vi "IO输入界面.vi"(8 "错误输入（无错误）":errorcluster, 10 "界面切换队列":refnum<queue>, 11 "VISA资源名称输入":refnum<visa-resource-name>) -> (0 "错误输出":errorcluster, 3 "VISA资源名称输出":refnum<visa-resource-name>)   [LabVIEW 2018]
panel:
  out "毫秒计时值":u32
  in  "枚举":T1(ring)
  in  "选项卡控件":enum32{"选项卡 1", "选项卡 2"}(tab)
  out "IO输出":bool
  out "X308-9#OK":bool
  out "?":bool
  out "?":bool
  out "X207-16#正在烧录":bool
  out "X206-15#正在烧录":bool
  out "X205-14#正在烧录":bool
  out "X204-13#正在烧录":bool
  out "X203-12#正在烧录":bool
  out "X202-11#正在烧录":bool
  out "X201-10#正在烧录":bool
  out "X200-9#正在烧录":bool
  out "X317-8#正在烧录":bool
  out "X316-7#正在烧录":bool
  out "X315-6#正在烧录":bool
  out "X314-5#正在烧录":bool
  out "X313-4#正在烧录":bool
  out "X312-3#正在烧录":bool
  out "X311-2#正在烧录":bool
  out "X310-1#正在烧录":bool
  out "X30F-16#OK":bool
  out "X30E-15#OK":bool
  out "X30D-14#OK":bool
  out "X30C-13#OK":bool
  out "X30B-12#OK":bool
  out "X30A-11#OK":bool
  out "X309-10#OK":bool
  out "X307-8#OK":bool
  out "X306-7#OK":bool
  out "X305-6#OK":bool
  out "X304-5#OK":bool
  out "X303-4#OK":bool
  out "X302-3#OK":bool
  out "X301-2#OK":bool
  out "X300-1#OK":bool
  out "X1F-Z2轴伺服报警":bool
  out "X1E-Z1轴伺服报警":bool
  out "X1D-Y轴伺服报警":bool
  out "X1C-X轴伺服报警":bool
  out "X1B":bool
  out "X1A":bool
  out "X19":bool
  out "X18":bool
  out "X17-2号真空达到":bool
  out "X16-1号真空到达":bool
  out "X15-手柄快慢切换":bool
  out "X14手柄Z1+":bool
  out "X13-手柄Z1-":bool
  out "X12-手柄X-":bool
  out "X11-手柄X+":bool
  out "X10-手柄Y+":bool
  out "XF-手柄Y-":bool
  out "XE":bool
  out "XD":bool
  out "XC-自动换盘完成":bool
  out "XB-卷带收料完成":bool
  out "XA-启动按钮":bool
  out "X9-紧急停止":bool
  out "X8-开门检测":bool
  out "X7-Z2原点":bool
  out "X6-Z1原点":bool
  out "X5-Y轴原点":bool
  out "X4-X轴原点":bool
  out "X3":bool
  out "X2":bool
  out "X1":bool
  out "DDT90356":dbl
  out "DDT90348":dbl
  out "自动界面":bool
  out "手动界面":bool
  out "参数界面":bool
  out "IO界面":bool
  out "产品界面":bool
  out "字符串":string
  out "DDT90352":dbl
  out "DDT90360":dbl
  out "通讯周期":dbl
  out "DT1184":T2(ring)
  out "X0":bool
  # "X"
  # "Z1"
  # "XXXXX自动化设备有限公司"
  # "Z2"
  # "Y"
  # "本\n体\n输\n入"
  # "扩\n展\n输\n入"
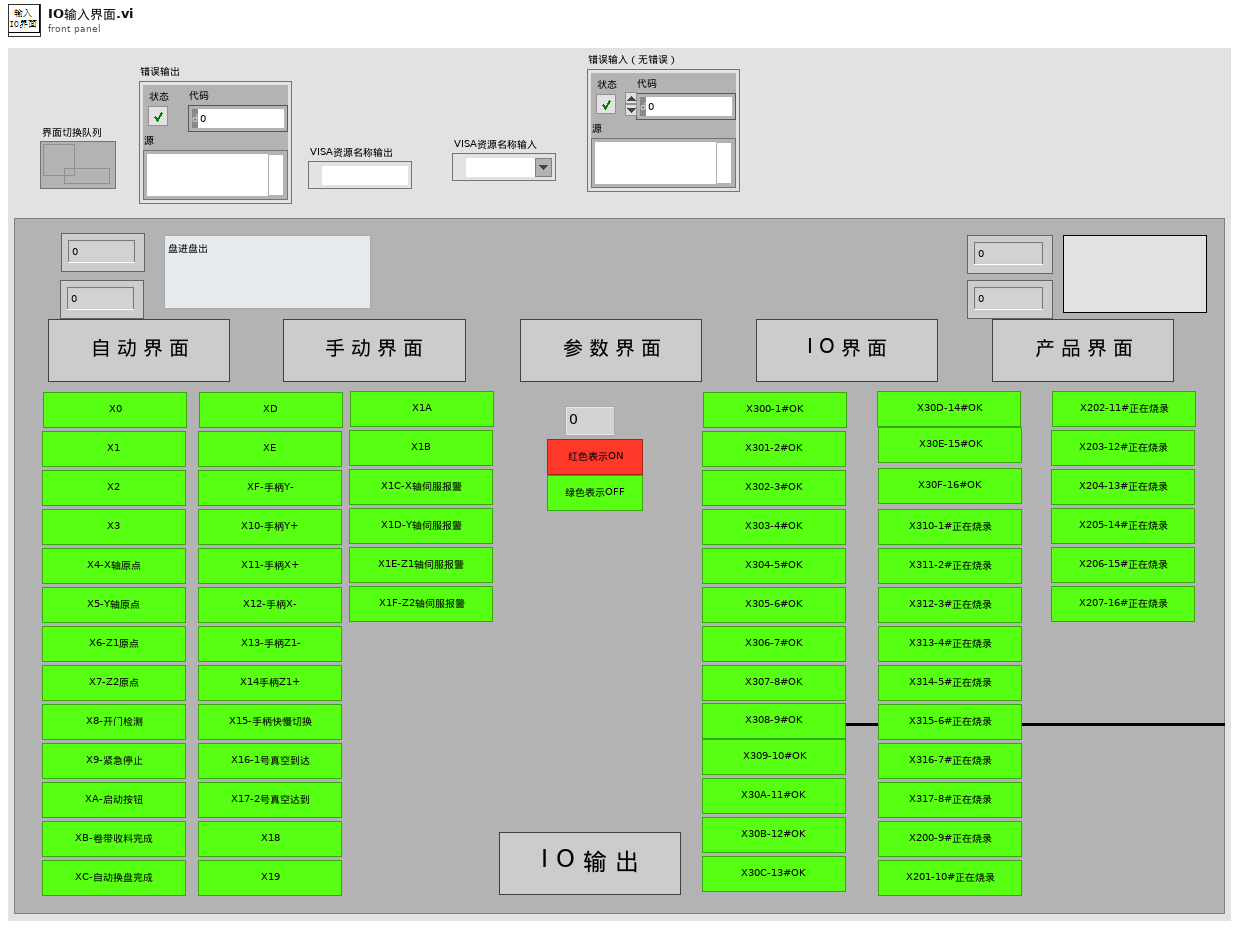
[diagram p1: front panel]
types:
  T1 = enum16{"读初始化", "读X310+8", "读X200+8", "读X308+8", "读X300+8", "读X18+8", "读X10+8", "读X8+8", "读X0+8", "读DDT90356", "读DT1184", "读DDT90348", ""}
  T2 = enum16{"盘进盘出", "卷进卷出", "盘进卷出", "管进盘出", "管进卷出", "卷进盘出", ""}
  T3 = enum8{"Enabled", "Disabled", "Disabled and Grayed Out"}
  T4 = typedef "数据簇.ctl" = cluster{"字符串":string, "数值":i32, "布尔":bool}
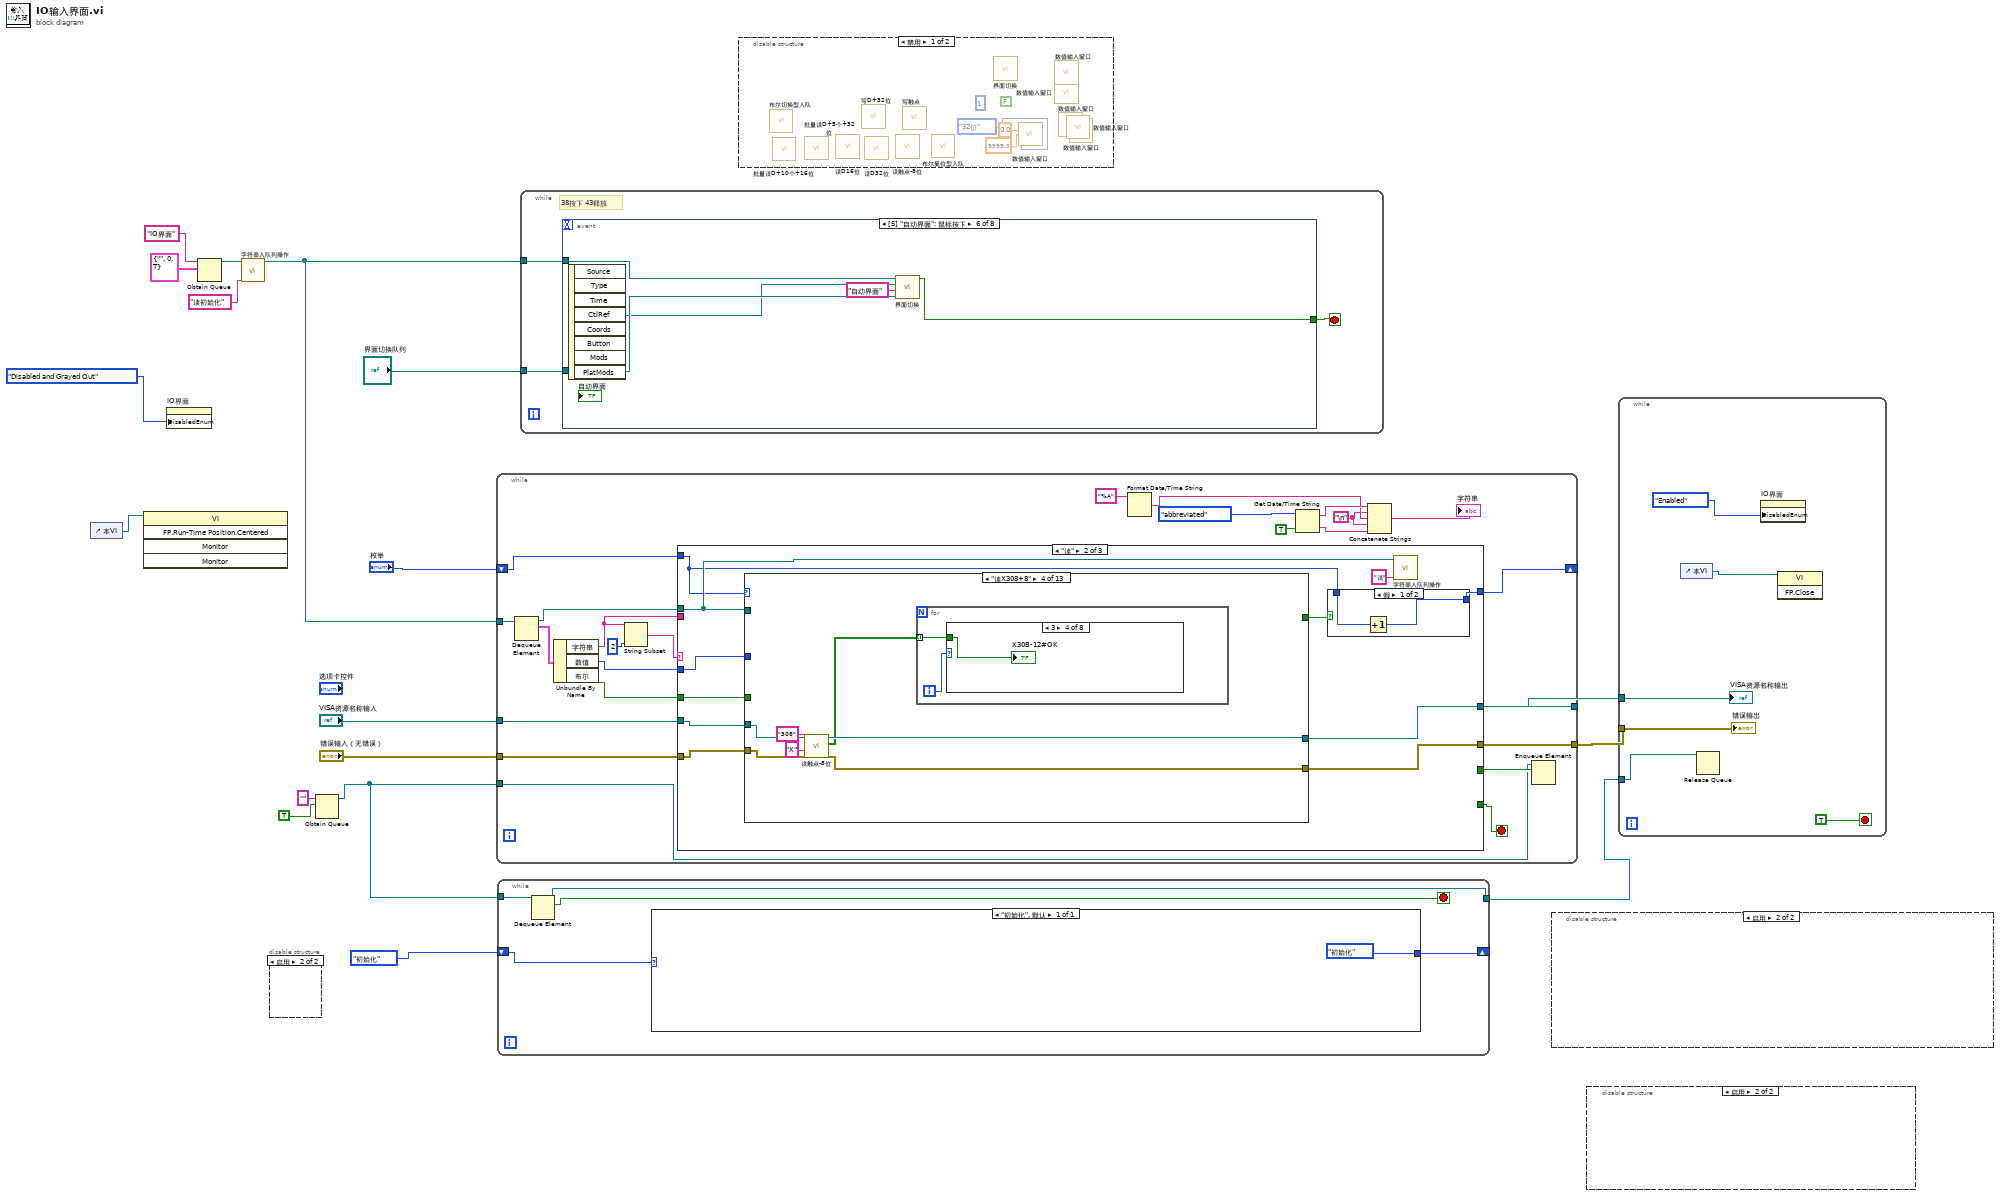
[diagram p0: block diagram]
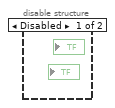
[diagram p2: hidden frame]
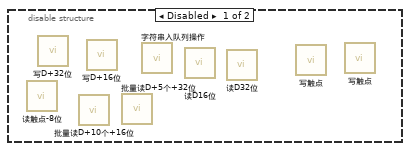
[diagram p20: hidden frame]
diagram:
  n1 = control-ref of="本VI"() -> (w1:refnum<vi>)
  n2 = invoke class="VI" method="FP.Run-Time Position.Centered"(reference=w1) -> ()  [unwired: 4 in, 5 out]
  n3 = property on="IO界面" class="Bool"("DisabledEnum"=T3."Disabled and Grayed Out" ("禁用")) -> ()  [unwired: 2 in, 2 out]
  n4 = Obtain Queue(name (unnamed)="IO界面" ("名称（未命名）"), element data type=T4 {"字符串"="", "数值"=0, "布尔"=TRUE}) -> (queue out=w11:refnum<queue>)  [unwired: 3 in, 2 out]
  n5 = call "字符串入队列操作.vi"("字符消息入队列"="读初始化", "界面切换队列"=w11) -> ("队列输出"=w3:refnum<queue>)  [unwired: 9 in]
  n6 = disable-structure shown="启用" {
    frame Disabled {
    }
    frame Enabled {
    }
  }
  n7 = Obtain Queue(name (unnamed)="" ("名称（未命名）"), element data type=TRUE) -> (queue out=w6:refnum<queue>)  [unwired: 3 in, 2 out]
  n8 = while {
    tunnel: w3 -> [w39]
    tunnel: "VISA资源名称输入" -> [w32]
    tunnel: "错误输入（无错误）" -> [w31]
    tunnel: [w30] -> w13
    tunnel: [w29] -> w12
    shift-right: [w26] -> _
    shift-left: "枚举" -> [w27]
    tunnel: w6 -> [w19]
    stop <- w21 stop-if-true
    w23 = "\n"
    n9 = Dequeue Element(queue=w39) -> (queue out=w36:refnum<queue>, element=w38:T4)  [unwired: 2 in, 2 out]
    n10 = Unbundle By Name(w38) -> ("字符串"=w33:string, "数值"=w35:i32, "布尔"=w34:bool)
    n11 = String Subset(string=w33, length (rest)=2 ("长度（剩余）")) -> (substring=w37:string)  [unwired: 1 in]
    n12 = case shown="\"读\"" w37 {
      selector: w37 -> [w46 _ _]
      tunnel: w36 -> [_ w54 w259]
      tunnel: w35 -> [_ w61 w258]
      tunnel: w34 -> [_ w60 w257]
      tunnel: w33 -> [_ _ w251]
      tunnel: w32 -> [w45 w59 w256]
      tunnel: w31 -> [w44 w58 w255]
      tunnel: [w45 w57 w253] -> w30
      tunnel: [w44 w56 w252] -> w29
      tunnel: [_ _ w254] -> w21
      tunnel: w27 -> [_ w52 _]
      tunnel: [_ w51 _] -> w26
      tunnel: [_ _ w249] -> w20
      frame "", Default {
        n13 = Concatenate Strings("无对应消息分支**" ("消息"), w46, "**" ("字符串"), "读写状态机" ("字符串")) -> (w48:string)
        n14 = One Button Dialog(message=w48) -> ()  [unwired: 1 in, 1 out]
      }
      frame "读" {
        n15 = case shown="\"读X308+8\"" w52 {
          tunnel: w54 -> [_ _ _ _ _ _ _ _ _ _ _ _ _]
          tunnel: w61 -> [_ _ _ _ _ _ _ _ _ _ _ _ _]
          tunnel: w59 -> [w66 w73 w90 w107 w124 w141 w158 w175 w192 w214 w223 w236 w248]
          tunnel: w58 -> [w65 w72 w89 w106 w123 w140 w157 w174 w191 w213 w222 w235 w247]
          tunnel: [w66 w69 w86 w103 w120 w139 w154 w171 w190 w212 w221 w234 w248] -> w57
          tunnel: [w65 w68 w85 w102 w119 w138 w153 w170 w189 w211 w220 w233 w247] -> w56
          tunnel: w60 -> [_ _ _ _ _ _ _ _ _ _ _ _ _]
          tunnel: [_ _ _ _ _ _ _ _ _ _ _ _ TRUE] -> w53
          frame "读初始化" {
            n16 = Tick Count (ms)() -> (millisecond timer value=→"毫秒计时值":u32)
          }
          frame "读X310+8" {
            n17 = call "读触点-8位.vi"("error out"=w72, "触点类型"="X", "读取起始地址"="310", "VISA resource name out"=w73) -> ("error IO"=w68:errorcluster, "读取布尔数组"=w67:bool[], "VISA resource name out 2"=w69:refnum<visa-resource-name>)  [unwired: 4 in, 1 out]
            n18 = for {
              tunnel: w67 -> [w74] mode=indexing
              i -> [w75]
              n19 = case shown="7" w75 {
                tunnel: w74 -> [w76 w77 w78 w79 w80 w81 w82 w83]
                frame 0, Default {
                  "X310-1#正在烧录" <- w76
                }
                frame 1 {
                  "X311-2#正在烧录" <- w77
                }
                frame 2 {
                  "X312-3#正在烧录" <- w78
                }
                frame 3 {
                  "X313-4#正在烧录" <- w79
                }
                frame 4 {
                  "X314-5#正在烧录" <- w80
                }
                frame 5 {
                  "X315-6#正在烧录" <- w81
                }
                frame 6 {
                  "X316-7#正在烧录" <- w82
                }
                frame 7 {
                  "X317-8#正在烧录" <- w83
                }
              }
            }
          }
          frame "读X200+8" {
            n20 = call "读触点-8位.vi"("error out"=w89, "触点类型"="X", "读取起始地址"="200", "VISA resource name out"=w90) -> ("error IO"=w85:errorcluster, "读取布尔数组"=w84:bool[], "VISA resource name out 2"=w86:refnum<visa-resource-name>)  [unwired: 4 in, 1 out]
            n21 = for {
              tunnel: w84 -> [w91] mode=indexing
              i -> [w92]
              n22 = case shown="7" w92 {
                tunnel: w91 -> [w93 w94 w95 w96 w97 w98 w99 w100]
                frame 0, Default {
                  "X200-9#正在烧录" <- w93
                }
                frame 1 {
                  "X201-10#正在烧录" <- w94
                }
                frame 2 {
                  "X202-11#正在烧录" <- w95
                }
                frame 3 {
                  "X203-12#正在烧录" <- w96
                }
                frame 4 {
                  "X204-13#正在烧录" <- w97
                }
                frame 5 {
                  "X205-14#正在烧录" <- w98
                }
                frame 6 {
                  "X206-15#正在烧录" <- w99
                }
                frame 7 {
                  "X207-16#正在烧录" <- w100
                }
              }
            }
          }
          frame "读X308+8" {
            n23 = call "读触点-8位.vi"("error out"=w106, "触点类型"="X", "读取起始地址"="308", "VISA resource name out"=w107) -> ("error IO"=w102:errorcluster, "读取布尔数组"=w101:bool[], "VISA resource name out 2"=w103:refnum<visa-resource-name>)  [unwired: 4 in, 1 out]
            n24 = for {
              tunnel: w101 -> [w108] mode=indexing
              i -> [w109]
              n25 = case shown="3" w109 {
                tunnel: w108 -> [w110 w111 w112 w113 w114 w115 w116 w117]
                frame 0, Default {
                  "X308-9#OK" <- w110
                }
                frame 1 {
                  "X309-10#OK" <- w111
                }
                frame 2 {
                  "X30A-11#OK" <- w112
                }
                frame 3 {
                  "X30B-12#OK" <- w113
                }
                frame 4 {
                  "X30C-13#OK" <- w114
                }
                frame 5 {
                  "X30D-14#OK" <- w115
                }
                frame 6 {
                  "X30E-15#OK" <- w116
                }
                frame 7 {
                  "X30F-16#OK" <- w117
                }
              }
            }
          }
          frame "读X300+8" {
            n26 = call "读触点-8位.vi"("error out"=w123, "触点类型"="X", "读取起始地址"="300", "VISA resource name out"=w124) -> ("error IO"=w119:errorcluster, "读取布尔数组"=w118:bool[], "VISA resource name out 2"=w120:refnum<visa-resource-name>)  [unwired: 4 in, 1 out]
            n27 = for {
              tunnel: w118 -> [w125] mode=indexing
              i -> [w126]
              n28 = case shown="7" w126 {
                tunnel: w125 -> [w127 w128 w129 w130 w131 w132 w133 w134]
                frame 0, Default {
                  "X300-1#OK" <- w127
                }
                frame 1 {
                  "X301-2#OK" <- w128
                }
                frame 2 {
                  "X302-3#OK" <- w129
                }
                frame 3 {
                  "X303-4#OK" <- w130
                }
                frame 4 {
                  "X304-5#OK" <- w131
                }
                frame 5 {
                  "X305-6#OK" <- w132
                }
                frame 6 {
                  "X306-7#OK" <- w133
                }
                frame 7 {
                  "X307-8#OK" <- w134
                }
              }
            }
          }
          frame "读X18+8" {
            n29 = call "读触点-8位.vi"("error out"=w140, "触点类型"="X", "读取起始地址"="18", "VISA resource name out"=w141) -> ("error IO"=w138:errorcluster, "读取布尔数组"=w135:bool[], "VISA resource name out 2"=w139:refnum<visa-resource-name>)  [unwired: 4 in, 1 out]
            n30 = for {
              tunnel: w135 -> [w142] mode=indexing
              i -> [w143]
              n31 = case shown="7" w143 {
                tunnel: w142 -> [w144 w145 w146 w147 w148 w149 w150 w151]
                frame 0, Default {
                  "X18" <- w144
                }
                frame 1 {
                  "X19" <- w145
                }
                frame 2 {
                  "X1A" <- w146
                }
                frame 3 {
                  "X1B" <- w147
                }
                frame 4 {
                  "X1C-X轴伺服报警" <- w148
                }
                frame 5 {
                  "X1D-Y轴伺服报警" <- w149
                }
                frame 6 {
                  "X1E-Z1轴伺服报警" <- w150
                }
                frame 7 {
                  "X1F-Z2轴伺服报警" <- w151
                }
              }
            }
          }
          frame "读X10+8" {
            n32 = call "读触点-8位.vi"("error out"=w157, "触点类型"="X", "读取起始地址"="10", "VISA resource name out"=w158) -> ("error IO"=w153:errorcluster, "读取布尔数组"=w152:bool[], "VISA resource name out 2"=w154:refnum<visa-resource-name>)  [unwired: 4 in, 1 out]
            n33 = for {
              tunnel: w152 -> [w159] mode=indexing
              i -> [w160]
              n34 = case shown="0, 默认" w160 {
                tunnel: w159 -> [w161 w162 w163 w164 w165 w166 w167 w168]
                frame 0, Default {
                  "X10-手柄Y+" <- w161
                }
                frame 1 {
                  "X11-手柄X+" <- w162
                }
                frame 2 {
                  "X12-手柄X-" <- w163
                }
                frame 3 {
                  "X13-手柄Z1-" <- w164
                }
                frame 4 {
                  "X14手柄Z1+" <- w165
                }
                frame 5 {
                  "X15-手柄快慢切换" <- w166
                }
                frame 6 {
                  "X16-1号真空到达" <- w167
                }
                frame 7 {
                  "X17-2号真空达到" <- w168
                }
              }
            }
          }
          frame "读X8+8" {
            n35 = call "读触点-8位.vi"("error out"=w174, "触点类型"="X", "读取起始地址"="8", "VISA resource name out"=w175) -> ("error IO"=w170:errorcluster, "读取布尔数组"=w169:bool[], "VISA resource name out 2"=w171:refnum<visa-resource-name>)  [unwired: 4 in, 1 out]
            n36 = for {
              tunnel: w169 -> [w176] mode=indexing
              i -> [w177]
              n37 = case shown="7" w177 {
                tunnel: w176 -> [w178 w179 w180 w181 w182 w183 w184 w185]
                frame 0, Default {
                  "X8-开门检测" <- w178
                }
                frame 1 {
                  "X9-紧急停止" <- w179
                }
                frame 2 {
                  "XA-启动按钮" <- w180
                }
                frame 3 {
                  "XB-卷带收料完成" <- w181
                }
                frame 4 {
                  "XC-自动换盘完成" <- w182
                }
                frame 5 {
                  "XD" <- w183
                }
                frame 6 {
                  "XE" <- w184
                }
                frame 7 {
                  "XF-手柄Y-" <- w185
                }
              }
            }
          }
          frame "读X0+8" {
            n38 = call "读触点-8位.vi"("error out"=w191, "触点类型"="X", "读取起始地址"="0", "VISA resource name out"=w192) -> ("error IO"=w189:errorcluster, "读取布尔数组"=w186:bool[], "VISA resource name out 2"=w190:refnum<visa-resource-name>)  [unwired: 4 in, 1 out]
            n39 = for {
              tunnel: w186 -> [w193] mode=indexing
              i -> [w194]
              n40 = case shown="7" w194 {
                tunnel: w193 -> [w195 w196 w197 w198 w199 w200 w201 w202]
                frame 0, Default {
                  "X0" <- w195
                }
                frame 1 {
                  "X1" <- w196
                }
                frame 2 {
                  "X2" <- w197
                }
                frame 3 {
                  "X3" <- w198
                }
                frame 4 {
                  "X4-X轴原点" <- w199
                }
                frame 5 {
                  "X5-Y轴原点" <- w200
                }
                frame 6 {
                  "X6-Z1原点" <- w201
                }
                frame 7 {
                  "X7-Z2原点" <- w202
                }
              }
            }
          }
          frame "读DDT90356" {
            n41 = call "批量读D+5个+32位.vi"("error out"=w213, "读取D地址"=90356, "VISA resource name out"=w214) -> ("error IO"=w211:errorcluster, "数组"=w217:i32[], "VISA resource name out 2"=w212:refnum<visa-resource-name>)  [unwired: 5 in, 1 out]
            n42 = Index Array(array=w217, index #1=0 ("索引"), index #2=2 ("索引")) -> (element #1=w210:i32, element #2=w209:i32)
            n43 = To Double Precision Float(number=w210) -> (double precision float=w208:dbl)
            n44 = To Double Precision Float(number=w209) -> (double precision float=w205:dbl)
            n45 = Divide(x=w208, y=100.0) -> (x/y=→"DDT90356":dbl)
            n46 = Divide(x=w205, y=100.0) -> (x/y=→"DDT90360":dbl)
          }
          frame "读DT1184" {
            n47 = call "读D16位.vi"("error out"=w222, "读取D地址"=1184, "VISA resource name out"=w223) -> ("error IO"=w220:errorcluster, "数值"=→"DT1184":u32, "VISA resource name out 2"=w221:refnum<visa-resource-name>)  [unwired: 5 in, 1 out]
          }
          frame "读DDT90348" {
            n48 = call "批量读D+5个+32位.vi"("error out"=w235, "读取D地址"=90348, "VISA resource name out"=w236) -> ("error IO"=w233:errorcluster, "数组"=w240:i32[], "VISA resource name out 2"=w234:refnum<visa-resource-name>)  [unwired: 5 in, 1 out]
            n49 = Index Array(array=w240, index #1=0 ("索引"), index #2=2 ("索引")) -> (element #1=w232:i32, element #2=w231:i32)
            n50 = To Double Precision Float(number=w231) -> (double precision float=w226:dbl)
            n51 = To Double Precision Float(number=w232) -> (double precision float=w230:dbl)
            n52 = Divide(x=w226, y=100.0) -> (x/y=→"DDT90352":dbl)
            n53 = Divide(x=w230, y=100.0) -> (x/y=→"DDT90348":dbl)
          }
          frame "" {
            n54 = local read "毫秒计时值"() -> (w244:u32)
            n55 = Tick Count (ms)() -> (millisecond timer value=w245:u32)
            n56 = Subtract(x=w245, y=w244) -> (x-y=w243:u32)
            n57 = Divide(x=w243, y=u32 1000) -> (x/y=→"通讯周期":dbl)
          }
        }
        n58 = case shown="假" w53 {
          tunnel: w52 -> [w63 _]
          tunnel: [w62 _] -> w51
          frame False {
            n59 = Increment(x=w63) -> (x+1=w62:T1)
          }
          frame True {
          }
        }
        n60 = call "字符串入队列操作.vi"("字符消息入队列"="读", "界面切换队列"=w54) -> ()  [unwired: 9 in, 1 out]
      }
      frame "写" {
        n61 = call "状态匹配.vi"("输入状态"=w251) -> ("输出状态"=w250:string)  [unwired: 10 in]
        n62 = case shown="\"写退出\"" w250 {
          selector: w250 -> [w262 _ _ _ _]
          tunnel: w259 -> [_ _ _ _ w302]
          tunnel: w258 -> [_ w268 w285 _ _]
          tunnel: w257 -> [_ _ _ w296 _]
          tunnel: w256 -> [w261 w278 w289 w301 w307]
          tunnel: w255 -> [w260 w277 w288 w300 w306]
          tunnel: [_ _ _ _ w305] -> w254
          tunnel: [w261 w276 w287 w299 w307] -> w253
          tunnel: [w260 w275 w286 w298 w306] -> w252
          tunnel: w251 -> [_ w267 w279 w290 _]
          tunnel: [_ _ _ _ w305] -> w249
          frame "", Default {
            n63 = Concatenate Strings("无对应消息分支**" ("消息"), w262, "**" ("字符串"), "写状态机" ("字符串")) -> (w266:string)
            n64 = One Button Dialog(message=w266) -> ()  [unwired: 1 in, 1 out]
          }
          frame "写DT" {
            n65 = String Length(string=w267) -> (length=w273:i32)
            n66 = Subtract(x=w273, y=4) -> (x-y=w271:i32)
            n67 = String Subset(string=w267, offset (0)=4 ("偏移量(0)"), length (rest)=w271) -> (substring=w270:string)
            n68 = Decimal String To Number(string=w270) -> (number=w269:i32)  [unwired: 2 in, 1 out]
            n69 = call "写D+16位.vi"("error out"=w277, "输入数值"=w268, "输入地址D"=w269, "VISA resource name out"=w278) -> ("error out 2"=w275:errorcluster, "VISA resource name out 2"=w276:refnum<visa-resource-name>)  [unwired: 3 in, 3 out]
          }
          frame "写DDT" {
            n70 = String Length(string=w279) -> (length=w283:i32)
            n71 = Subtract(x=w283, y=5) -> ()  [unwired: 1 out]
            n72 = String Subset(string=w279, offset (0)=5 ("偏移量(0)")) -> (substring=w280:string)  [unwired: 1 in]
            n73 = Decimal String To Number(string=w280) -> (number=w281:i32)  [unwired: 2 in, 1 out]
            n74 = call "写D+32位.vi"("error out"=w288, "输入数值"=w285, "输入地址D"=w281, "VISA resource name out"=w289) -> ("error out 2"=w286:errorcluster, "VISA resource name out 2"=w287:refnum<visa-resource-name>)  [unwired: 4 in, 2 out]
          }
          frame "写R" {
            n75 = String Length(string=w290) -> (length=w294:i32)
            n76 = Subtract(x=w294, y=3) -> (x-y=w292:i32)
            n77 = String Subset(string=w290, offset (0)=3 ("偏移量(0)"), length (rest)=w292) -> (substring=w291:string)
            n78 = call "写触点.vi"("布尔"=w296, "error out"=w300, "触点类型"="R", "写入起始地址"=w291, "VISA resource name out"=w301) -> ("error IO"=w298:errorcluster, "VISA resource name out 2"=w299:refnum<visa-resource-name>)  [unwired: 4 in, 1 out]
          }
          frame "写退出" {
            w305 = TRUE
            n79 = Flush Queue(queue=w302) -> (queue out=w303:refnum<queue>, error out=w304:errorcluster)  [unwired: 1 in, 1 out]
            n80 = Release Queue(queue=w303, error in (no error)=w304) -> ()  [unwired: 1 in, 3 out]
          }
        }
      }
    }
    n81 = Format Date/Time String(time format string (%c)="%A" ("时间格式字符串(%c)")) -> (date/time string=w24:string)  [unwired: 2 in]
    n82 = Get Date/Time String(date format (0)=enum16{"short", "long", "abbreviated"}."abbreviated" ("日期格式(0)"), want seconds? (F)=TRUE ("需要秒？(F)")) -> (date string=w41:string, time string=w22:string)  [unwired: 1 in]
    n83 = Concatenate Strings(w41, w23, w24, w23, w22) -> (→"字符串":string)
    n84 = Enqueue Element(queue=w19, element=w20) -> ()  [unwired: 2 in, 3 out]
  }
  n85 = while {
    shift-right: [w311] -> _
    shift-left: enum16{"初始化"}."初始化" -> [w312]
    tunnel: w6 -> [w310]
    tunnel: [w308] -> w5
    stop <- w309 stop-if-true
    n86 = Dequeue Element(queue=w310) -> (queue out=w308:refnum<queue>, element=w309:bool)  [unwired: 2 in, 2 out]
    n87 = case shown="\"初始化\", 默认" w312 {
      tunnel: [enum16{"初始化"}."初始化"] -> w311
      frame "初始化", Default {
      }
    }
  }
  n88 = while {
    tunnel: w3 -> [w315]
    tunnel: "界面切换队列" -> [w314]
    stop <- w316 stop-if-true
    # "38按下 43释放"
    n89 = event shown="[5] \"自动界面\": 鼠标按下" {
      selector: _ -> [_ _ _ _ _ _ _ _]
      dyn-events: _ -> [_ _ _ _ _ _ _ _]
      timeout: _ -> [_ _ _ _ _ _ _ _]
      tunnel: [w317 w322 w327 w332 w337 w342 _ w349] -> w316
      tunnel: w315 -> [w321 w326 w331 w336 w341 w346 _ w348]
      tunnel: w314 -> [w320 w325 w330 w335 w340 w345 _ w347]
      event "IO界面": Mouse Down {
        n90 = event-data() -> ("CtlRef"=w319:refnum<vi>)  [unwired: 1 in, 7 out]
        n91 = call "界面切换.vi"("界面切换队列输入"=w320, "切换界面名称输入"="IO界面", "Bool引用句柄"=w319, "状态转移输入"=w321) -> ("布尔"=w317:bool)  [unwired: 7 in]
      }
      event "IO输出": Mouse Down {
        n92 = event-data() -> ("CtlRef"=w324:refnum<vi>)  [unwired: 1 in, 7 out]
        n93 = call "界面切换.vi"("界面切换队列输入"=w325, "切换界面名称输入"="IO输出界面", "Bool引用句柄"=w324, "状态转移输入"=w326) -> ("布尔"=w322:bool)  [unwired: 7 in]
      }
      event "参数界面": Mouse Down {
        n94 = event-data() -> ("CtlRef"=w328:refnum<vi>)  [unwired: 1 in, 7 out]
        n95 = call "界面切换.vi"("界面切换队列输入"=w330, "切换界面名称输入"="参数界面", "Bool引用句柄"=w328, "状态转移输入"=w331) -> ("布尔"=w327:bool)  [unwired: 7 in]
      }
      event "产品界面": Mouse Down {
        n96 = event-data() -> ("CtlRef"=w334:refnum<vi>)  [unwired: 1 in, 7 out]
        n97 = call "界面切换.vi"("界面切换队列输入"=w335, "切换界面名称输入"="产品界面", "Bool引用句柄"=w334, "状态转移输入"=w336) -> ("布尔"=w332:bool)  [unwired: 7 in]
      }
      event "手动界面": Mouse Down {
        n98 = event-data() -> ("CtlRef"=w339:refnum<vi>)  [unwired: 1 in, 7 out]
        n99 = call "界面切换.vi"("界面切换队列输入"=w340, "切换界面名称输入"="手动界面", "Bool引用句柄"=w339, "状态转移输入"=w341) -> ("布尔"=w337:bool)  [unwired: 7 in]
      }
      event "自动界面": Mouse Down {
        n100 = event-data() -> ("CtlRef"=w344:refnum<vi>)  [unwired: 1 in, 7 out]
        n101 = call "界面切换.vi"("界面切换队列输入"=w345, "切换界面名称输入"="自动界面", "Bool引用句柄"=w344, "状态转移输入"=w346) -> ("布尔"=w342:bool)  [unwired: 7 in]
      }
      event Timeout {
        n102 = event-data() -> ()  [unwired: 1 in, 3 out]
      }
      event Panel Close? {
        n103 = event-data() -> ()  [unwired: 1 in, 4 out]
        n104 = Two Button Dialog(message="确定退出程序？" ("消息")) -> (T button?=w350:bool)  [unwired: 2 in]
        n105 = case shown="真" w350 {
          tunnel: [_ TRUE] -> w349
          tunnel: w348 -> [_ w355]
          tunnel: w347 -> [_ w354]
          frame False {
          }
          frame True {
            n106 = call "字符串入队列操作.vi"("字符消息入队列"="退出", "界面切换队列"=w354) -> ()  [unwired: 9 in, 1 out]
            n107 = call "字符串入队列操作.vi"("字符消息入队列"="写退出", "界面切换队列"=w355) -> ()  [unwired: 9 in, 1 out]
          }
        }
        n108 = event-data("Discard?"=TRUE ("放弃？")) -> ()  [unwired: 1 in, 1 out]
      }
    }
  }
  n109 = disable-structure shown="禁用" {
    frame Disabled {
      (unwired) u32 1 ("转换比例")
      (unwired) FALSE ("忽略数值上下限")
      n110 = call "布尔切换型入队.vi"() -> ()  [unwired: 12 in]
      n111 = call "批量读D+10个+16位.vi"() -> ()  [unwired: 8 in, 4 out]
      n112 = call "批量读D+5个+32位.vi"() -> ()  [unwired: 8 in, 4 out]
      n113 = call "读D16位.vi"() -> ()  [unwired: 8 in, 4 out]
      n114 = call "写D+32位.vi"() -> ()  [unwired: 8 in, 4 out]
      n115 = call "读D32位.vi"() -> ()  [unwired: 9 in, 3 out]
      n116 = call "读触点-8位.vi"() -> ()  [unwired: 8 in, 4 out]
      n117 = call "写触点.vi"() -> ()  [unwired: 9 in, 3 out]
      n118 = call "布尔复位型入队.vi"() -> ()  [unwired: 8 in, 2 out]
      n119 = call "界面切换.vi"() -> ()  [unwired: 11 in, 1 out]
      n120 = call "数值输入窗口.vi"("输入下限"=0.0, "输入上限"=9999.0, "数据类型"=enum16{"32位", "16位"}."32位") -> ("转换比例"=w361:u32)  [unwired: 9 in, 3 out]
      n121 = call "数值输入窗口.vi"() -> ()  [unwired: 13 in, 3 out]
      n122 = call "数值输入窗口.vi"() -> ()  [unwired: 13 in, 3 out]
      n123 = call "数值输入窗口.vi"() -> ()  [unwired: 13 in, 3 out]
      n124 = call "数值输入窗口.vi"() -> ()  [unwired: 13 in, 3 out]
      n125 = call "数值输入窗口.vi"() -> ()  [unwired: 13 in, 3 out]
    }
    frame Enabled {
    }
  }
  n126 = disable-structure shown="启用" {
    frame Disabled {
      n127 = for {
        i -> [w363]
        n128 = case shown="9" w363 {
          frame 0, Default {
          }
          frame 1 {
          }
          frame 2 {
          }
          frame 3 {
          }
          frame 4 {
          }
          frame 5 {
          }
          frame 6 {
          }
          frame 7 {
          }
          frame 8 {
          }
          frame 9 {
          }
        }
      }
      n129 = for {
        i -> [w362]
        n130 = case shown="1" w362 {
          frame 0, Default {
          }
          frame 1 {
          }
          frame 2 {
          }
          frame 3 {
          }
          frame 4 {
          }
          frame 5 {
          }
          frame 6 {
          }
          frame 7 {
          }
        }
      }
    }
    frame Enabled {
    }
  }
  n131 = disable-structure shown="启用" {
    frame Disabled {
      n132 = call "读触点-8位.vi"() -> ()  [unwired: 8 in, 4 out]
      n133 = call "写D+32位.vi"() -> ()  [unwired: 8 in, 4 out]
      n134 = call "批量读D+10个+16位.vi"() -> ()  [unwired: 8 in, 4 out]
      n135 = call "写D+16位.vi"() -> ()  [unwired: 7 in, 5 out]
      n136 = call "批量读D+5个+32位.vi"() -> ()  [unwired: 8 in, 4 out]
      n137 = call "字符串入队列操作.vi"() -> ()  [unwired: 11 in, 1 out]
      n138 = call "读D16位.vi"() -> ()  [unwired: 8 in, 4 out]
      n139 = call "读D32位.vi"() -> ()  [unwired: 9 in, 3 out]
      n140 = call "写触点.vi"() -> ()  [unwired: 9 in, 3 out]
      n141 = call "写触点.vi"() -> ()  [unwired: 9 in, 3 out]
    }
    frame Enabled {
    }
  }
  n142 = while {
    tunnel: w13 -> [w368]
    tunnel: w12 -> [w367]
    tunnel: w5 -> [w366]
    stop <- TRUE stop-if-true
    n143 = control-ref of="本VI"() -> (w364:refnum<vi>)
    n144 = Release Queue(queue=w366) -> ()  [unwired: 2 in, 3 out]
    n145 = property on="IO界面" class="Bool"("DisabledEnum"=T3."Enabled" ("禁用")) -> ()  [unwired: 2 in, 2 out]
    n146 = invoke class="VI" method="FP.Close"(reference=w364) -> ()  [unwired: 2 in, 3 out]
    "VISA资源名称输出" <- w368
    "错误输出" <- w367
  }
